vi "总程序.vi"() -> ()   [LabVIEW 2015]
uses:
  idd.vi
  global1.vi
  <vilib>/Utility/file.llb/Write To Spreadsheet File (DBL).vi
  <vilib>/gmath/NI_Gmath.lvlib
  <vilib>/measure/NI_MABase.lvlib
panel:
  in  "机构复位":bool
  in  "数据清零":bool
  in  "数据保存":bool
  in  "启动":bool
  out "实时曲线":dbl(graph)
  out "试验数据曲线":cluster{dbl[], dbl[]}[](graph)
  in  "Numeric 4":i32
  out "e3 2":dbl
  out "e2 2":dbl
  out "Numeric 2":i32
  in  "a 2":dbl=0.62
  in  "times 2":i32=1 min=1 max=100
  out "V0  2":dbl
  out "e3 3":dbl
  out "e2 3":dbl
  out "Numeric 3":i32
  out "V0  3":dbl
  in  "a 3":dbl=0.65
  in  "times 3":i32=1 min=1 max=100
  out "Numeric":i32
  out "e2":dbl
  out "e3":dbl
  out "V0":dbl
  in  "a":dbl=0.5
  in  "times":i32=1 min=1 max=100
  in  "ChoiseCards 3":i32
  out "hDevice 3":u32 format="%x"
  out "idd(szout) 3":u32[](array[numeric])
  in  "ChoiseCards 2":i32
  out "hDevice 2":u32 format="%x"
  out "idd(szout) 2":u32[](array[numeric])
  out "hDevice(out)":i32 format="%x"
  in  "DA通道":i32=1
  in  "DAData":i32=1024
  in  "ChoiseCards":i32
  out "hDevice":u32 format="%x"
  out "idd(szout)":u32[](array[numeric])
  in  "Tab Control":enum32{"阶跃", "正弦", "方波"}(tab)
  out "实际位移":dbl
  in  "采样开始":bool
  in  "采样周期":u8(knob) scale=0.0..50.0
  in  "比例系数":dbl
  in  "积分系数":dbl
  in  "目标位移":dbl=150.0
  in  "DA通道":i32=1 min=0 max=1
  in  "AD通道":i32=14 min=0 max=31
  in  "微分系数":dbl
  in  "采样次数":i32=600
  in  "采样开始3":bool
  in  "采样周期":u8(knob) scale=0.0..50.0
  in  "周期(s)":dbl=5.0
  in  "中心(mm)":dbl=100.0
  in  "幅值(mm)":dbl=50.0
  in  "微分系数 3":dbl
  in  "积分系数 3":dbl
  in  "比例系数 3":dbl
  in  "采样次数 3":i32=400
  in  "AD通道 3":i32=14 min=0 max=31
  in  "DA通道 5":i32=1 min=0 max=1
  in  "采样开始2":bool
  in  "采样周期":u8(knob) scale=0.0..50.0
  in  "占空比":dbl=50.0 format="%0.2f"
  in  "目标位移2":dbl=100.0
  in  "目标位移1":dbl=150.0
  in  "微分系数 2":dbl
  in  "积分系数 2":dbl
  in  "比例系数 2":dbl
  in  "采样次数 2":i32=800
  in  "AD通道 2":i32=14 min=0 max=31
  in  "DA通道 3":i32=1 min=0 max=1
  # "直流伺服电机位置控制实验台"
  # "PID控制器"
  # "PID控制器"
  # "PID控制器"
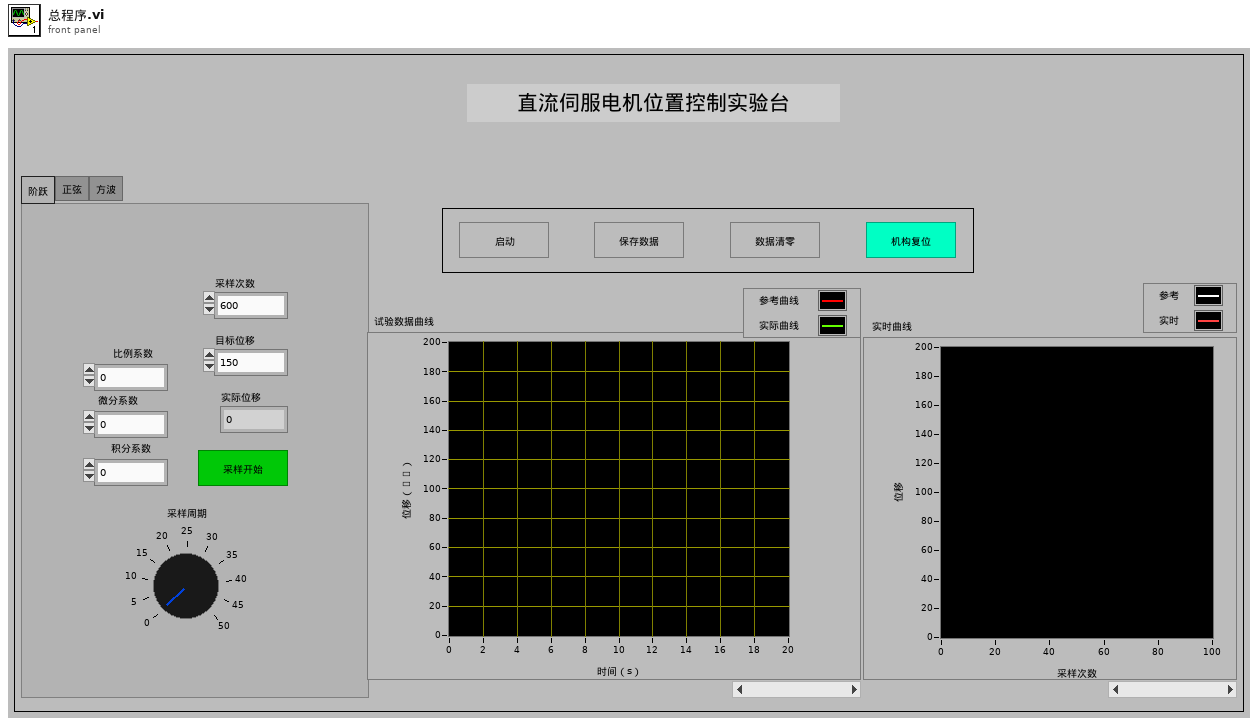
[diagram p1: front panel]
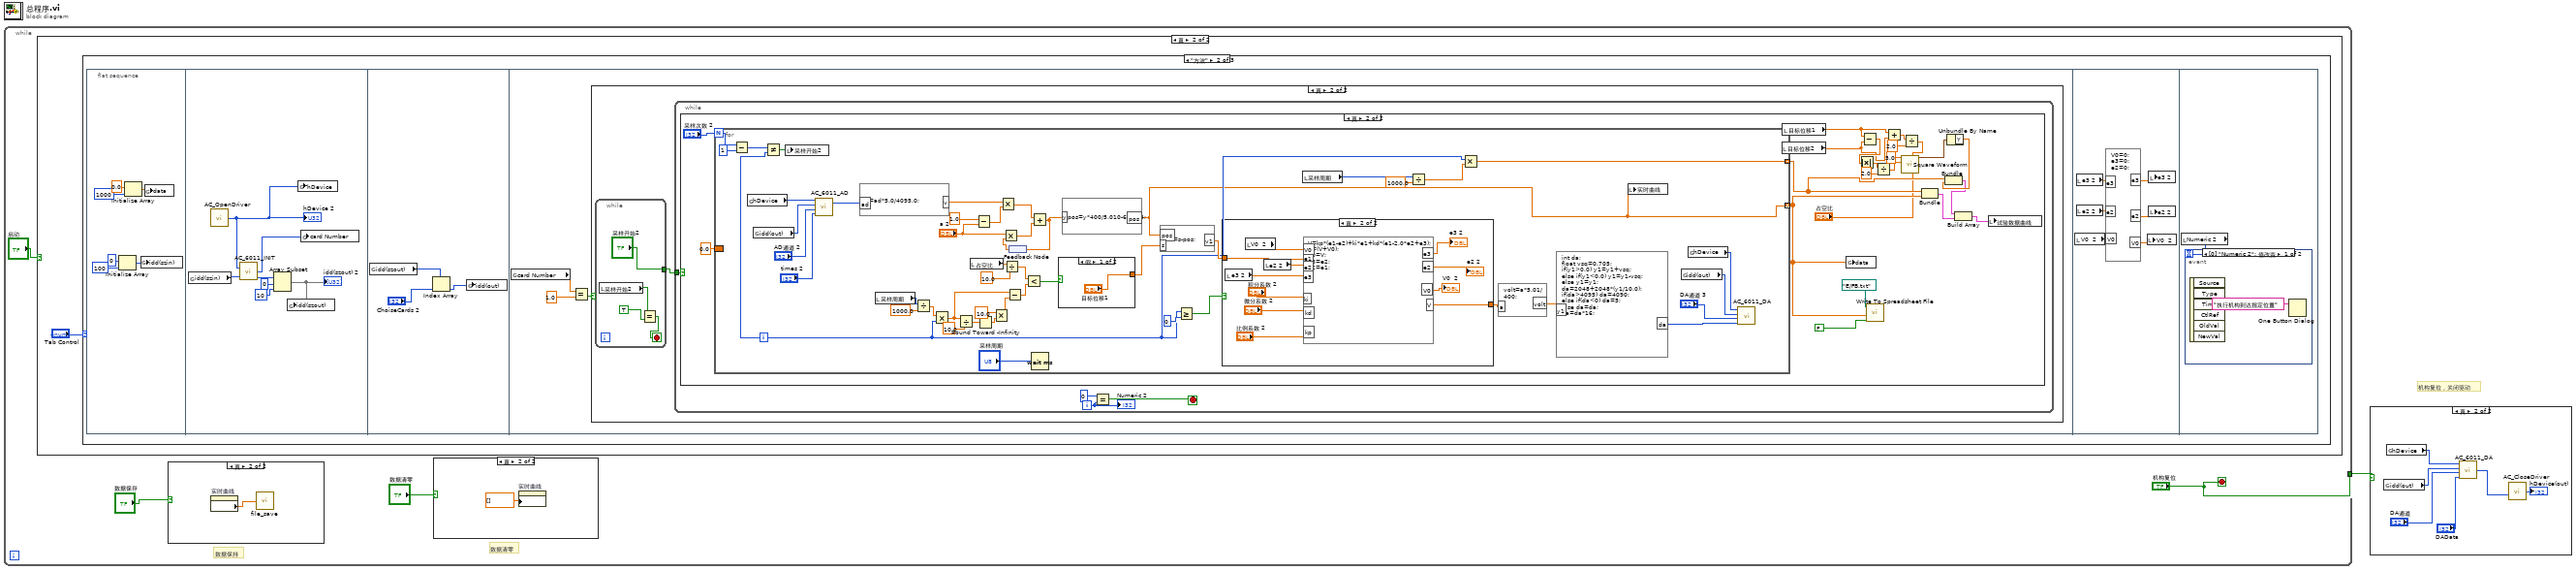
[diagram p0: block diagram]
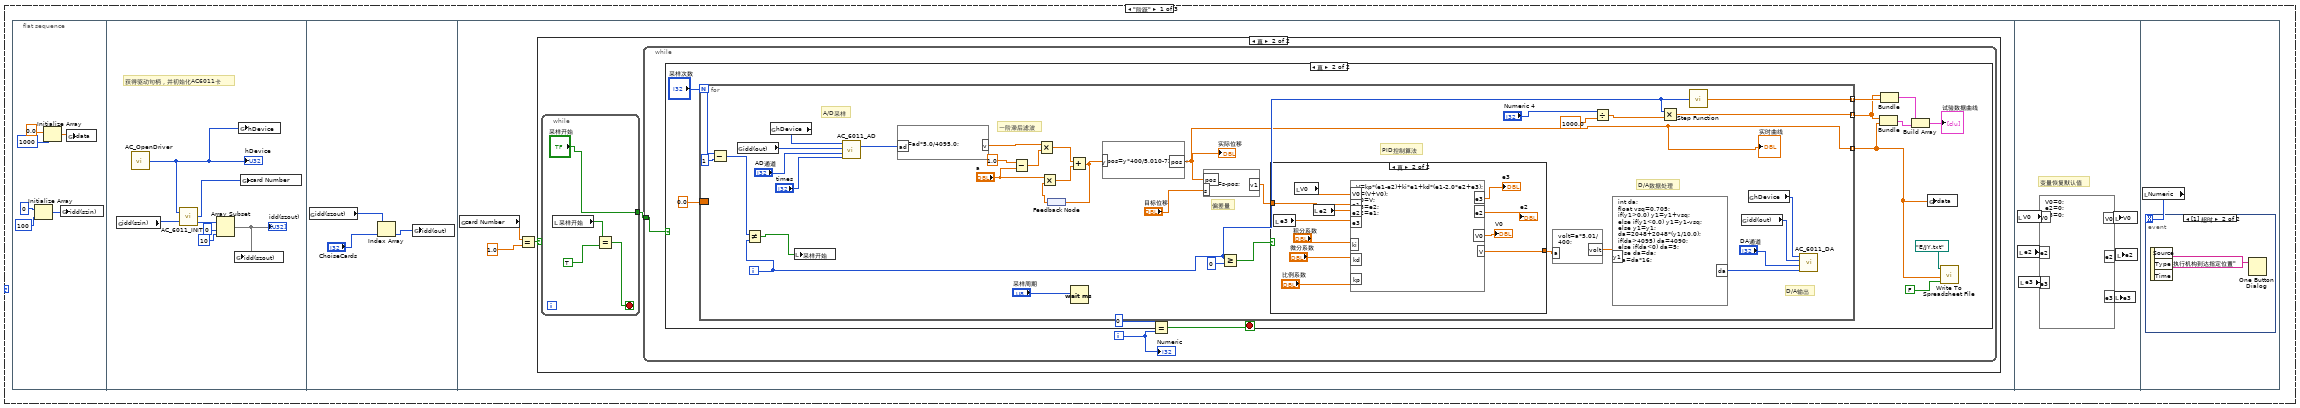
[diagram p6: hidden frame]
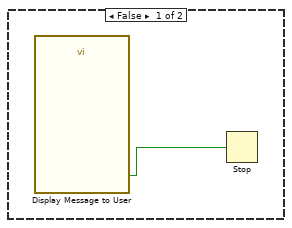
[diagram p7: hidden frame]
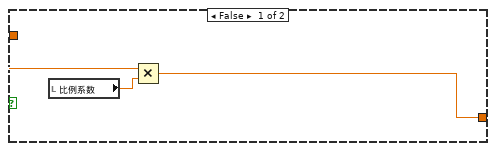
[diagram p9: hidden frame]
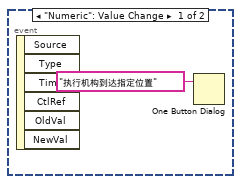
[diagram p10: hidden frame]
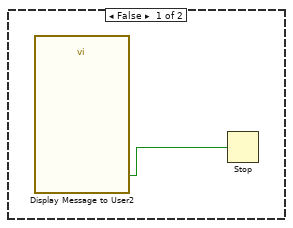
[diagram p11: hidden frame]
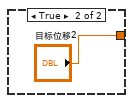
[diagram p13: hidden frame]
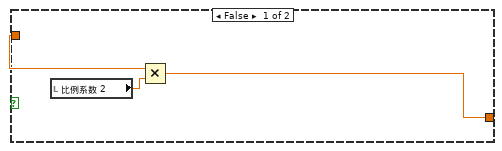
[diagram p14: hidden frame]
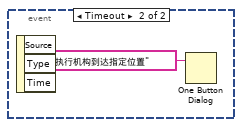
[diagram p15: hidden frame]
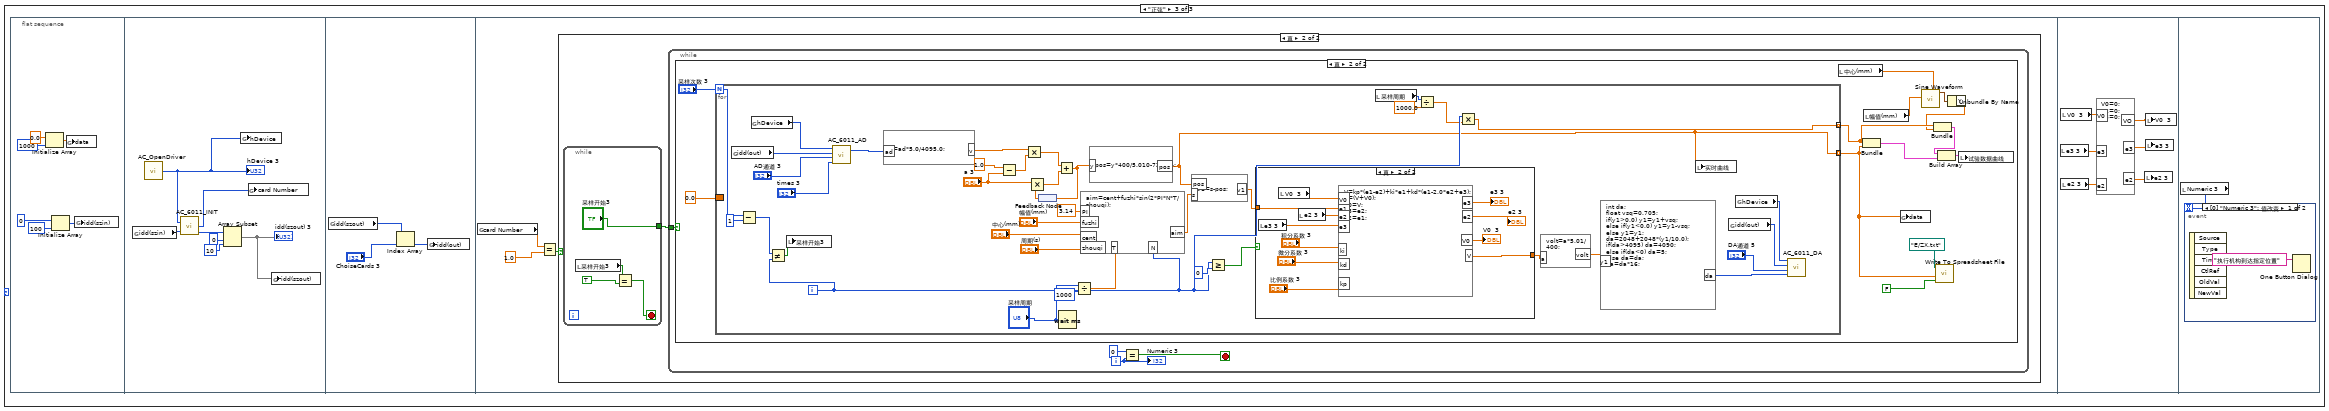
[diagram p16: hidden frame]
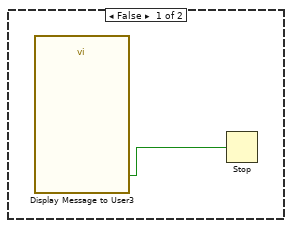
[diagram p17: hidden frame]
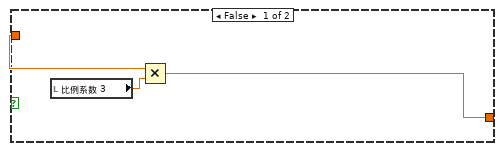
[diagram p19: hidden frame]
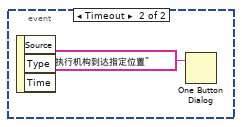
[diagram p20: hidden frame]
diagram:
  # "机构复位，关闭驱动"
  n1 = while {
    tunnel: ["机构复位"] -> w1
    stop <- "机构复位" stop-if-true
    # "数据清零"
    # "数据保持"
    n2 = case shown="真" "启动" {
      frame False {
      }
      frame True {
        n3 = case shown="\"方波\"" "Tab Control" {
          frame "阶跃" {
            n4 = flat-sequence {
              frame #0 {
                n5 = Initialize Array(0, 100) -> (w14:i32[])
                n6 = Initialize Array(0.0 ("element"), 1000 ("dimension size")) -> (w9:dbl[])
                n7 = global write "idd.vi" "idd(szin)"(w14) -> ()
                n8 = global write "global1.vi" "data"(w9) -> ()
              }
              frame #1 {
                # "获得驱动句柄，并初始化AC6011卡"
                n9 = global read "idd.vi" "idd(szin)"() -> (w17:u32[])
                n10 = call "AC_OpenDriver.vi"() -> ("hDevice"=w16:u32)  [unwired: 1 in]
                "hDevice" <- w16
                n11 = call "AC_6011_INIT.vi"("hDevice(in)"=w16, "idd(szin)"=w17) -> ("Cardc"=w15:i32, "idd(szout)"=w18:u32[])  [unwired: 1 out]
                n12 = Array Subset(array=w18, index=0, length=10) -> (w21:u32[])
                "idd(szout)" <- w21
                n13 = global write "idd.vi" "idd(szout)"(w21) -> ()
                n14 = global write "idd.vi" "hDevice"(w16) -> ()
                n15 = global write "global1.vi" "card Number"(w15) -> ()
              }
              frame #2 {
                n16 = global read "idd.vi" "idd(szout)"() -> (w24:u32[])
                n17 = Index Array "Index Array"(array=w24, index="ChoiseCards") -> (element=w22:u32)
                n18 = global write "idd.vi" "idd(out)"(w22) -> ()
              }
              frame #3 {
                n19 = global read "global1.vi" "card Number"() -> (w27:dbl)
                n20 = Equal?(x=w27, y=1.0) -> (x = y?=w25:bool)
                n21 = case shown="真" w25 {
                  frame False {
                    n22 = call "Display Message to User"() -> ("OK"=w28:bool)  [unwired: 10 in, 1 out]
                    n23 = Stop(stop? (T)=w28) -> ()
                  }
                  frame True {
                    n24 = while {
                      tunnel: ["采样开始"] -> w29
                      stop <- w32 stop-if-true
                      n25 = local read "采样开始"() -> (w30:bool)
                      n26 = Equal?(x=w30, y=TRUE) -> (x = y?=w32:bool)
                    }
                    n27 = while {
                      tunnel: w29 -> [w35]
                      i -> [w37]
                      stop <- w34 stop-if-true
                      n28 = case shown="真" w35 {
                        frame False {
                        }
                        frame True {
                          n29 = for {
                            N: "采样次数" -> [w59]
                            tunnel: [w48] -> w42 mode=indexing
                            tunnel: [w49] -> w44 mode=indexing
                            tunnel: [w50] -> w43 mode=indexing
                            border: 0.0 -> [_]
                            i -> [w56]
                            # "A/D采样"
                            # "偏差量"
                            # "一阶滞后滤波"
                            # "PID控制算法"
                            # "D/A输出"
                            # "D/A数据处理"
                            n30 = Subtract(x=w59, y=1) -> (x-y=w57:i32)
                            n31 = global read "idd.vi" "idd(out)"() -> (w80:u32)
                            n32 = Not Equal?(x=w57, y=w56) -> (x != y?=w52:bool)
                            n33 = global read "idd.vi" "hDevice"() -> (w79:u32)
                            n34 = local write "采样开始"(w52) -> ()
                            n35 = call "AC_6011_AD.vi"("times"="times", "ch"="AD通道", "idd(out)"=w80, "hDevice(in)"=w79) -> ("data"=w60:i32)  [unwired: 1 out]
                            n36 = formula code="v=ad*5.0/4095.0;"("ad"=w60) -> ("v"=w73:dbl)
                            n37 = Subtract(x=1.0, y="a") -> (x-y=w76:dbl)
                            n38 = Multiply(x=w73, y=w76) -> (x*y=w78:dbl)
                            n39 = feedback #1() -> (w65:dbl)
                            n40 = Multiply(x="a", y=w65) -> (x*y=w77:dbl)
                            n41 = Add(x=w78, y=w77) -> (x+y=w66:dbl)
                            n42 = feedback-in #1(w66) -> ()
                            n43 = Wait (ms)(milliseconds to wait="采样周期") -> ()  [unwired: 1 out]
                            n44 = formula code="pos=y*400/5.010-72.894;"("y"=w66) -> ("pos"=w48:dbl)
                            "实际位移" <- w48
                            "实时曲线" <- w48
                            n45 = formula code="v1=s-pos;"("pos"=w48, "s"="目标位移") -> ("v1"=w62:dbl)
                            n46 = Greater Or Equal?(x=w56, y=0) -> (x >= y?=w67:bool)
                            n47 = case shown="真" w67 {
                              tunnel: w62 -> [w85 w93]
                              tunnel: [w84 w92] -> w64
                              frame False {
                                n48 = local read "比例系数"() -> (w83:dbl)
                                n49 = Multiply(x=w85, y=w83) -> (x*y=w84:dbl)
                              }
                              frame True {
                                n50 = local read "e3"() -> (w87:dbl)
                                n51 = local read "V0"() -> (w90:dbl)
                                n52 = local read "e2"() -> (w86:dbl)
                                n53 = formula code="V=kp*(e1-e2)+ki*e1+kd*(e1-2.0*e2+e3);\nV=(V+V0);\nV0=V;\ne3=e2;\ne2=e1;"("e1"=w93, "e2"=w86, "e3"=w87, "ki"="积分系数", "kd"="微分系数", "kp"="比例系数", "V0"=w90) -> ("V"=w92:dbl, "V0"=→"V0":dbl, "e2"=→"e2":dbl, "e3"=→"e3":dbl)
                              }
                            }
                            n54 = formula code="volt=a*5.01/400;"("a"=w64) -> ("volt"=w63:dbl)
                            n55 = Divide(x="Numeric 4", y=1000.0) -> (x/y=w53:dbl)
                            n56 = formula code="int da;\nfloat vsq=0.705;\nif(y1>0.0) y1=y1+vsq;\nelse if(y1<0.0) y1=y1-vsq;\nelse y1=y1;\nda=2048+2048*(y1/10.0);\nif(da>4095) da=4090;\nelse if(da<0) da=5;\nelse da=da;\nda=da*16;"("y1"=w63) -> ("da"=w69:i32)
                            n57 = Multiply(x=w56, y=w53) -> (x*y=w50:dbl)
                            n58 = call <vilib>:"Step Function.vi"("x"=w56) -> ("step(x)"=w49:dbl)
                            n59 = global read "idd.vi" "idd(out)"() -> (w72:u32)
                            n60 = global read "idd.vi" "hDevice"() -> (w70:u32)
                            n61 = call "AC_6011_DA.vi"("DAData"=w69, "DAch"="DA通道", "idd(out)"=w72, "hDevice"=w70) -> ()  [unwired: 1 out]
                          }
                          n62 = Bundle(w43, w42) -> (w40:cluster{dbl[], dbl[]})  [unwired: 1 in]
                          n63 = Bundle(w43, w44) -> (w41:cluster{dbl[], dbl[]})  [unwired: 1 in]
                          n64 = Build Array(w41, w40) -> (→"试验数据曲线":cluster{dbl[], dbl[]}[])
                          n65 = global write "global1.vi" "data"(w42) -> ()
                          n66 = call-poly <vilib>:"Write To Spreadsheet File.vi"("append to file? (new file:F)"=FALSE, "1D data"=w42, "file path (dialog if empty)"=path "E:/JY.txt") -> ()  [unwired: 5 in, 1 out]
                        }
                      }
                      n67 = Equal?(x=0, y=w37) -> (x = y?=w34:bool)
                      "Numeric" <- w37
                    }
                  }
                }
              }
              frame #4 {
                # "变量恢复默认值"
                n68 = local read "V0"() -> (w97:dbl)
                n69 = local read "e2"() -> (w99:dbl)
                n70 = local read "e3"() -> (w101:dbl)
                n71 = formula code="V0=0;\ne2=0;\ne3=0;"("V0"=w97, "e2"=w99, "e3"=w101) -> ("V0"=w98:dbl, "e2"=w100:dbl, "e3"=w102:dbl)
                n72 = local write "V0"(w98) -> ()
                n73 = local write "e3"(w102) -> ()
                n74 = local write "e2"(w100) -> ()
              }
              frame #5 {
                n75 = local read "Numeric"() -> (w103:i32)
                n76 = event shown="[1] 超时" {
                  selector: _ -> [_ _]
                  dyn-events: _ -> [_ _]
                  timeout: w103 -> [_ _]
                  event "Numeric": Value Change {
                    n77 = event-data() -> ()  [unwired: 1 in, 6 out]
                    n78 = One Button Dialog(message="执行机构到达指定位置") -> ()  [unwired: 1 in, 1 out]
                  }
                  event Timeout {
                    n79 = event-data() -> ()  [unwired: 1 in, 3 out]
                    n80 = One Button Dialog(message="执行机构到达指定位置") -> ()  [unwired: 1 in, 1 out]
                  }
                }
              }
            }
          }
          frame "方波" {
            n81 = flat-sequence {
              frame #0 {
                n82 = Initialize Array(0, 100) -> (w111:i32[])
                n83 = Initialize Array(0.0 ("element"), 1000 ("dimension size")) -> (w106:dbl[])
                n84 = global write "idd.vi" "idd(szin)"(w111) -> ()
                n85 = global write "global1.vi" "data"(w106) -> ()
              }
              frame #1 {
                n86 = global read "idd.vi" "idd(szin)"() -> (w114:u32[])
                n87 = call "AC_OpenDriver.vi"() -> ("hDevice"=w113:u32)  [unwired: 1 in]
                "hDevice 2" <- w113
                n88 = call "AC_6011_INIT.vi"("hDevice(in)"=w113, "idd(szin)"=w114) -> ("Cardc"=w112:i32, "idd(szout)"=w115:u32[])  [unwired: 1 out]
                n89 = Array Subset(array=w115, index=0, length=10) -> (w118:u32[])
                "idd(szout) 2" <- w118
                n90 = global write "idd.vi" "idd(szout)"(w118) -> ()
                n91 = global write "idd.vi" "hDevice"(w113) -> ()
                n92 = global write "global1.vi" "card Number"(w112) -> ()
              }
              frame #2 {
                n93 = global read "idd.vi" "idd(szout)"() -> (w121:u32[])
                n94 = Index Array "Index Array"(array=w121, index="ChoiseCards 2") -> (element=w119:u32)
                n95 = global write "idd.vi" "idd(out)"(w119) -> ()
              }
              frame #3 {
                n96 = global read "global1.vi" "card Number"() -> (w124:dbl)
                n97 = Equal?(x=w124, y=1.0) -> (x = y?=w122:bool)
                n98 = case shown="真" w122 {
                  frame False {
                    n99 = call "Display Message to User2"() -> ("OK"=w125:bool)  [unwired: 10 in, 1 out]
                    n100 = Stop(stop? (T)=w125) -> ()
                  }
                  frame True {
                    n101 = while {
                      tunnel: ["采样开始2"] -> w126
                      stop <- w129 stop-if-true
                      n102 = local read "采样开始2"() -> (w128:bool)
                      n103 = Equal?(x=w128, y=TRUE) -> (x = y?=w129:bool)
                    }
                    n104 = while {
                      tunnel: w126 -> [w131]
                      i -> [w134]
                      stop <- w132 stop-if-true
                      n105 = case shown="真" w131 {
                        frame False {
                        }
                        frame True {
                          n106 = for {
                            N: "采样次数 2" -> [w169]
                            tunnel: [w161] -> w152 mode=indexing
                            tunnel: [w182] -> w149 mode=indexing
                            border: 0.0 -> [_]
                            i -> [w167]
                            n107 = Subtract(x=w169, y=1) -> (x-y=w166:i32)
                            n108 = global read "idd.vi" "hDevice"() -> (w201:u32)
                            n109 = global read "idd.vi" "idd(out)"() -> (w202:u32)
                            n110 = Not Equal?(x=w166, y=w167) -> (x != y?=w160:bool)
                            n111 = local write "采样开始2"(w160) -> ()
                            n112 = call "AC_6011_AD.vi"("times"="times 2", "ch"="AD通道 2", "idd(out)"=w202, "hDevice(in)"=w201) -> ("data"=w183:i32)  [unwired: 1 out]
                            n113 = formula code="v=ad*5.0/4095.0;"("ad"=w183) -> ("v"=w195:dbl)
                            n114 = local read "采样周期"() -> (w157:u8)
                            n115 = Divide(x=w157, y=1000.0) -> (x/y=w159:dbl)
                            n116 = Multiply(x=w159, y=w167) -> (x*y=w173:dbl)
                            n117 = Divide(x=w173, y=10.0) -> (x/y=w174:dbl)
                            n118 = local read "占空比"() -> (w176:dbl)
                            n119 = Subtract(x=1.0, y="a 2") -> (x-y=w198:dbl)
                            n120 = Round Toward -Infinity(1:w174) -> (0:w179:dbl)
                            n121 = Multiply(x=10.0, y=w179) -> (x*y=w177:dbl)
                            n122 = Multiply(x=w195, y=w198) -> (x*y=w200:dbl)
                            n123 = Divide(x=w176, y=10.0) -> (x/y=w171:dbl)
                            n124 = Subtract(x=w173, y=w177) -> (x-y=w170:dbl)
                            n125 = feedback #2() -> (w187:dbl)
                            n126 = Multiply(x="a 2", y=w187) -> (x*y=w199:dbl)
                            n127 = Less?(x=w171, y=w170) -> (x < y?=w172:bool)
                            n128 = Add(x=w200, y=w199) -> (x+y=w188:dbl)
                            n129 = feedback-in #2(w188) -> ()
                            n130 = Wait (ms)(milliseconds to wait="采样周期") -> ()  [unwired: 1 out]
                            n131 = case shown="假" w172 {
                              tunnel: ["目标位移1" "目标位移2"] -> w181
                              frame False {
                              }
                              frame True {
                              }
                            }
                            n132 = formula code="pos=y*400/5.010-68.864;"("y"=w188) -> ("pos"=w161:dbl)
                            n133 = formula code="v1=s-pos;"("pos"=w161, "s"=w181) -> ("v1"=w184:dbl)
                            n134 = Greater Or Equal?(x=w167, y=0) -> (x >= y?=w189:bool)
                            n135 = case shown="真" w189 {
                              tunnel: w184 -> [w209 w217]
                              tunnel: [w208 w216] -> w186
                              frame False {
                                n136 = local read "比例系数 2"() -> (w207:dbl)
                                n137 = Multiply(x=w209, y=w207) -> (x*y=w208:dbl)
                              }
                              frame True {
                                n138 = local read "e3 2"() -> (w211:dbl)
                                n139 = local read "V0  2"() -> (w214:dbl)
                                n140 = local read "e2 2"() -> (w210:dbl)
                                n141 = formula code="V=kp*(e1-e2)+ki*e1+kd*(e1-2.0*e2+e3);\nV=(V+V0);\nV0=V;\ne3=e2;\ne2=e1;"("e1"=w217, "e2"=w210, "e3"=w211, "ki"="积分系数 2", "kd"="微分系数 2", "kp"="比例系数 2", "V0"=w214) -> ("V"=w216:dbl, "V0"=→"V0  2":dbl, "e2"=→"e2 2":dbl, "e3"=→"e3 2":dbl)
                              }
                            }
                            n142 = local read "采样周期"() -> (w162:u8)
                            n143 = Divide(x=w162, y=1000.0) -> (x/y=w163:dbl)
                            n144 = Multiply(x=w167, y=w163) -> (x*y=w182:dbl)
                            n145 = formula code="volt=a*5.01/400;"("a"=w186) -> ("volt"=w185:dbl)
                            n146 = formula code="int da;\nfloat vsq=0.705;\nif(y1>0.0) y1=y1+vsq;\nelse if(y1<0.0) y1=y1-vsq;\nelse y1=y1;\nda=2048+2048*(y1/10.0);\nif(da>4095) da=4090;\nelse if(da<0) da=5;\nelse da=da;\nda=da*16;"("y1"=w185) -> ("da"=w191:i32)
                            n147 = local write "实时曲线"(w161) -> ()
                            n148 = global read "idd.vi" "idd(out)"() -> (w194:u32)
                            n149 = global read "idd.vi" "hDevice"() -> (w192:u32)
                            n150 = call "AC_6011_DA.vi"("DAData"=w191, "DAch"="DA通道 3", "idd(out)"=w194, "hDevice"=w192) -> ()  [unwired: 1 out]
                          }
                          n151 = local read "目标位移2"() -> (w144:dbl)
                          n152 = local read "目标位移1"() -> (w145:dbl)
                          n153 = global write "global1.vi" "data"(w152) -> ()
                          n154 = Subtract(x=w145, y=w144) -> (x-y=w151:dbl)
                          n155 = Absolute Value(x=w151) -> (abs(x)=w139:dbl)
                          n156 = call-poly <vilib>:"Write To Spreadsheet File.vi"("append to file? (new file:F)"=FALSE, "1D data"=w152, "file path (dialog if empty)"=path "E:/FB.txt") -> ()  [unwired: 5 in, 1 out]
                          n157 = Divide(x=w139, y=2.0) -> (x/y=w138:dbl)
                          n158 = Add(x=w145, y=w144) -> (x+y=w142:dbl)
                          n159 = Divide(x=w142, y=2.0) -> (x/y=w141:dbl)
                          n160 = call <vilib>:"Square Waveform.vi"("duty cycle (%)"="占空比", "offset"=w141, "amplitude"=w138, "frequency"=5.0) -> ("signal out"=w150:waveform(dbl))  [unwired: 6 in, 1 out]
                          n161 = Bundle(w149, w152) -> (w146:cluster{dbl[], dbl[]})  [unwired: 1 in]
                          n162 = Unbundle By Name(w150) -> ("Y"=w148:dbl[])
                          n163 = Bundle(w149, "Y"=w148) -> (w147:cluster{dbl[], "Y":dbl[]})  [unwired: 1 in]
                          n164 = Build Array(w147, w146) -> (w135:cluster{dbl[], "Y":dbl[]}[])
                          n165 = local write "试验数据曲线"(w135) -> ()
                        }
                      }
                      n166 = Equal?(x=0, y=w134) -> (x = y?=w132:bool)
                      "Numeric 2" <- w134
                    }
                  }
                }
              }
              frame #4 {
                n167 = local read "V0  2"() -> (w225:dbl)
                n168 = local read "e3 2"() -> (w221:dbl)
                n169 = local read "e2 2"() -> (w223:dbl)
                n170 = formula code="V0=0;\ne3=0;\ne2=0;"("e3"=w221, "e2"=w223, "V0"=w225) -> ("e3"=w222:dbl, "e2"=w224:dbl, "V0"=w226:dbl)
                n171 = local write "V0  2"(w226) -> ()
                n172 = local write "e3 2"(w222) -> ()
                n173 = local write "e2 2"(w224) -> ()
              }
              frame #5 {
                n174 = local read "Numeric 2"() -> (w227:i32)
                n175 = event shown="[0] \"Numeric 2\": 值改变" {
                  selector: _ -> [_ _]
                  dyn-events: _ -> [_ _]
                  timeout: w227 -> [_ _]
                  event "Numeric 2": Value Change {
                    n176 = event-data() -> ()  [unwired: 1 in, 6 out]
                    n177 = One Button Dialog(message="执行机构到达指定位置") -> ()  [unwired: 1 in, 1 out]
                  }
                  event Timeout {
                    n178 = event-data() -> ()  [unwired: 1 in, 3 out]
                    n179 = One Button Dialog(message="执行机构到达指定位置") -> ()  [unwired: 1 in, 1 out]
                  }
                }
              }
            }
          }
          frame "正弦" {
            n180 = flat-sequence {
              frame #0 {
                n181 = Initialize Array(0.0 ("element"), 1000 ("dimension size")) -> (w230:dbl[])
                n182 = Initialize Array(0, 100) -> (w235:i32[])
                n183 = global write "global1.vi" "data"(w230) -> ()
                n184 = global write "idd.vi" "idd(szin)"(w235) -> ()
              }
              frame #1 {
                n185 = global read "idd.vi" "idd(szin)"() -> (w238:u32[])
                n186 = call "AC_OpenDriver.vi"() -> ("hDevice"=w237:u32)  [unwired: 1 in]
                "hDevice 3" <- w237
                n187 = call "AC_6011_INIT.vi"("hDevice(in)"=w237, "idd(szin)"=w238) -> ("Cardc"=w236:i32, "idd(szout)"=w239:u32[])  [unwired: 1 out]
                n188 = Array Subset(array=w239, index=0, length=10) -> (w242:u32[])
                "idd(szout) 3" <- w242
                n189 = global write "idd.vi" "hDevice"(w237) -> ()
                n190 = global write "global1.vi" "card Number"(w236) -> ()
                n191 = global write "idd.vi" "idd(szout)"(w242) -> ()
              }
              frame #2 {
                n192 = global read "idd.vi" "idd(szout)"() -> (w245:u32[])
                n193 = Index Array "Index Array"(array=w245, index="ChoiseCards 3") -> (element=w243:u32)
                n194 = global write "idd.vi" "idd(out)"(w243) -> ()
              }
              frame #3 {
                n195 = global read "global1.vi" "card Number"() -> (w248:dbl)
                n196 = Equal?(x=w248, y=1.0) -> (x = y?=w246:bool)
                n197 = case shown="真" w246 {
                  frame False {
                    n198 = call "Display Message to User3"() -> ("OK"=w249:bool)  [unwired: 10 in, 1 out]
                    n199 = Stop(stop? (T)=w249) -> ()
                  }
                  frame True {
                    n200 = while {
                      tunnel: ["采样开始3"] -> w250
                      stop <- w253 stop-if-true
                      n201 = local read "采样开始3"() -> (w252:bool)
                      n202 = Equal?(x=w252, y=TRUE) -> (x = y?=w253:bool)
                    }
                    n203 = while {
                      tunnel: w250 -> [w255]
                      i -> [w258]
                      stop <- w256 stop-if-true
                      n204 = case shown="真" w255 {
                        frame False {
                        }
                        frame True {
                          n205 = for {
                            N: "采样次数 3" -> [w281]
                            tunnel: [w272] -> w267 mode=indexing
                            tunnel: [w282] -> w263 mode=indexing
                            border: 0.0 -> [_]
                            i -> [w279]
                            n206 = global read "idd.vi" "idd(out)"() -> (w309:u32)
                            n207 = Subtract(x=w281, y=1) -> (x-y=w278:i32)
                            n208 = global read "idd.vi" "hDevice"() -> (w308:u32)
                            n209 = Not Equal?(x=w278, y=w279) -> (x != y?=w273:bool)
                            n210 = local write "采样开始3"(w273) -> ()
                            n211 = call "AC_6011_AD.vi"("times"="times 3", "ch"="AD通道 3", "idd(out)"=w309, "hDevice(in)"=w308) -> ("data"=w290:i32)  [unwired: 1 out]
                            n212 = formula code="v=ad*5.0/4095.0;"("ad"=w290) -> ("v"=w302:dbl)
                            n213 = Subtract(x=1.0, y="a 3") -> (x-y=w305:dbl)
                            n214 = Multiply(x=w302, y=w305) -> (x*y=w307:dbl)
                            n215 = feedback #3() -> (w294:dbl)
                            n216 = Multiply(x="a 3", y=w294) -> (x*y=w306:dbl)
                            n217 = Add(x=w307, y=w306) -> (x+y=w295:dbl)
                            n218 = feedback-in #3(w295) -> ()
                            n219 = Wait (ms)(milliseconds to wait="采样周期") -> ()  [unwired: 1 out]
                            n220 = Divide(x="采样周期", y=u32 1000) -> (x/y=w283:dbl)
                            n221 = formula code="aim=cent+fuzhi*sin(2*PI*N*T/zhouqi);"("N"=w279, "PI"=3.14 ("input variable"), "fuzhi"="幅值(mm)", "cent"="中心(mm)", "zhouqi"="周期(s)", "T"=w283) -> ("aim"=w289:dbl)
                            n222 = formula code="pos=y*400/5.010-72.894;"("y"=w295) -> ("pos"=w272:dbl)
                            n223 = formula code="v1=s-pos;"("pos"=w272, "s"=w289) -> ("v1"=w291:dbl)
                            n224 = Greater Or Equal?(x=w279, y=0) -> (x >= y?=w296:bool)
                            n225 = case shown="真" w296 {
                              tunnel: w291 -> [w314 w322]
                              tunnel: [w313 w321] -> w293
                              frame False {
                                n226 = local read "比例系数 3"() -> (w312:dbl)
                                n227 = Multiply(x=w314, y=w312) -> (x*y=w313:dbl)
                              }
                              frame True {
                                n228 = local read "e3 3"() -> (w316:dbl)
                                n229 = local read "V0  3"() -> (w319:dbl)
                                n230 = local read "e2 3"() -> (w315:dbl)
                                n231 = formula code="V=kp*(e1-e2)+ki*e1+kd*(e1-2.0*e2+e3);\nV=(V+V0);\nV0=V;\ne3=e2;\ne2=e1;"("e1"=w322, "e2"=w315, "e3"=w316, "ki"="积分系数 3", "kd"="微分系数 3", "kp"="比例系数 3", "V0"=w319) -> ("V"=w321:dbl, "V0"=→"V0  3":dbl, "e2"=→"e2 3":dbl, "e3"=→"e3 3":dbl)
                              }
                            }
                            n232 = local read "采样周期"() -> (w275:u8)
                            n233 = Divide(x=w275, y=1000.0) -> (x/y=w274:dbl)
                            n234 = Multiply(x=w279, y=w274) -> (x*y=w282:dbl)
                            n235 = formula code="volt=a*5.01/400;"("a"=w293) -> ("volt"=w292:dbl)
                            n236 = formula code="int da;\nfloat vsq=0.705;\nif(y1>0.0) y1=y1+vsq;\nelse if(y1<0.0) y1=y1-vsq;\nelse y1=y1;\nda=2048+2048*(y1/10.0);\nif(da>4095) da=4090;\nelse if(da<0) da=5;\nelse da=da;\nda=da*16;"("y1"=w292) -> ("da"=w298:i32)
                            n237 = local write "实时曲线"(w272) -> ()
                            n238 = global read "idd.vi" "idd(out)"() -> (w301:u32)
                            n239 = global read "idd.vi" "hDevice"() -> (w299:u32)
                            n240 = call "AC_6011_DA.vi"("DAData"=w298, "DAch"="DA通道 5", "idd(out)"=w301, "hDevice"=w299) -> ()  [unwired: 1 out]
                          }
                          n241 = local read "中心(mm)"() -> (w265:dbl)
                          n242 = Bundle(w263, w267) -> (w260:cluster{dbl[], dbl[]})  [unwired: 1 in]
                          n243 = local read "幅值(mm)"() -> (w266:dbl)
                          n244 = global write "global1.vi" "data"(w267) -> ()
                          n245 = call <vilib>:"Sine Waveform.vi"("offset"=w265, "amplitude"=w266) -> ("signal out"=w264:waveform(dbl))  [unwired: 8 in, 1 out]
                          n246 = call-poly <vilib>:"Write To Spreadsheet File.vi"("append to file? (new file:F)"=FALSE, "1D data"=w267, "file path (dialog if empty)"=path "E:/ZX.txt") -> ()  [unwired: 5 in, 1 out]
                          n247 = Unbundle By Name(w264) -> ("Y"=w262:dbl[])
                          n248 = Bundle(w263, "Y"=w262) -> (w261:cluster{dbl[], "Y":dbl[]})  [unwired: 1 in]
                          n249 = Build Array(w261, w260) -> (w259:cluster{dbl[], "Y":dbl[]}[])
                          n250 = local write "试验数据曲线"(w259) -> ()
                        }
                      }
                      n251 = Equal?(x=0, y=w258) -> (x = y?=w256:bool)
                      "Numeric 3" <- w258
                    }
                  }
                }
              }
              frame #4 {
                n252 = local read "e3 3"() -> (w328:dbl)
                n253 = local read "V0  3"() -> (w326:dbl)
                n254 = local read "e2 3"() -> (w329:dbl)
                n255 = formula code="V0=0;\ne2=0;\ne3=0;"("V0"=w326, "e3"=w328, "e2"=w329) -> ("VO"=w327:dbl, "e3"=w330:dbl, "e2"=w331:dbl)
                n256 = local write "e2 3"(w331) -> ()
                n257 = local write "V0  3"(w327) -> ()
                n258 = local write "e3 3"(w330) -> ()
              }
              frame #5 {
                n259 = local read "Numeric 3"() -> (w332:i32)
                n260 = event shown="[0] \"Numeric 3\": 值改变" {
                  selector: _ -> [_ _]
                  dyn-events: _ -> [_ _]
                  timeout: w332 -> [_ _]
                  event "Numeric 3": Value Change {
                    n261 = event-data() -> ()  [unwired: 1 in, 6 out]
                    n262 = One Button Dialog(message="执行机构到达指定位置") -> ()  [unwired: 1 in, 1 out]
                  }
                  event Timeout {
                    n263 = event-data() -> ()  [unwired: 1 in, 3 out]
                    n264 = One Button Dialog(message="执行机构到达指定位置") -> ()  [unwired: 1 in, 1 out]
                  }
                }
              }
            }
          }
        }
      }
    }
    n265 = case shown="真" "数据保存" {
      frame False {
      }
      frame True {
        n266 = property on="实时曲线" class="WFChart (严格)"() -> ("History Data"=w7:dbl[])  [unwired: 2 in, 2 out]
        n267 = call "file_save.vi"("Array"=w7) -> ()
      }
    }
    n268 = case shown="真" "数据清零" {
      frame False {
      }
      frame True {
        n269 = property on="实时曲线" class="WFChart (严格)"("History Data"=dbl[] []) -> ()  [unwired: 2 in, 2 out]
      }
    }
  }
  n270 = case shown="真" w1 {
    frame False {
    }
    frame True {
      n271 = global read "idd.vi" "idd(out)"() -> (w339:u32)
      n272 = global read "idd.vi" "hDevice"() -> (w340:u32)
      n273 = call "AC_6011_DA.vi"("DAData"="DAData", "DAch"="DA通道", "idd(out)"=w339, "hDevice"=w340) -> ("hDevice(out)"=w335:i32)
      n274 = call "AC_CloseDriver.vi"("hDevice(in)"=w335) -> ("hDevice(out)"=→"hDevice(out)":u32)
    }
  }
